vi "BSC simple.vi"() -> (0 "error out":errorcluster)   [LabVIEW 2016]
uses:
  C:/Users/Administrator/Downloads/LabVIEW/Kinesis/DLL Libraries/Thorlabs.MotionControl.Controls.dll
  DLL Libraries/Thorlabs.MotionControl.Controls.dll
  C:/Program Files (x86)/National Instruments/LabVIEW 2015/instr.lib/nLight Instruments/Motion Controller/Specific Models/Thorlabs Kinesis/Thorlabs.MotionControl.GenericMotorCLI.dll
  Program Files (x86)/National Instruments/LabVIEW 2015/instr.lib/nLight Instruments/Motion Controller/Specific Models/Thorlabs Kinesis/Thorlabs.MotionControl.GenericMotorCLI.dll
  C:/Program Files (x86)/National Instruments/LabVIEW 2015/instr.lib/nLight Instruments/Motion Controller/Specific Models/Thorlabs Kinesis/Thorlabs.MotionControl.Benchtop.StepperMotorCLI.dll
  Program Files (x86)/National Instruments/LabVIEW 2015/instr.lib/nLight Instruments/Motion Controller/Specific Models/Thorlabs Kinesis/Thorlabs.MotionControl.Benchtop.StepperMotorCLI.dll
panel:
  out "Position":dbl
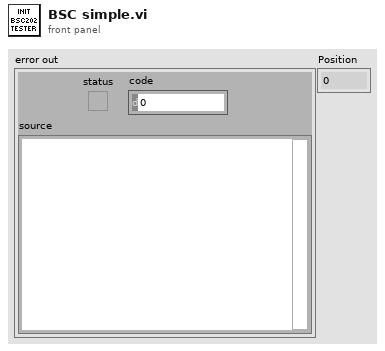
[diagram p1: front panel]
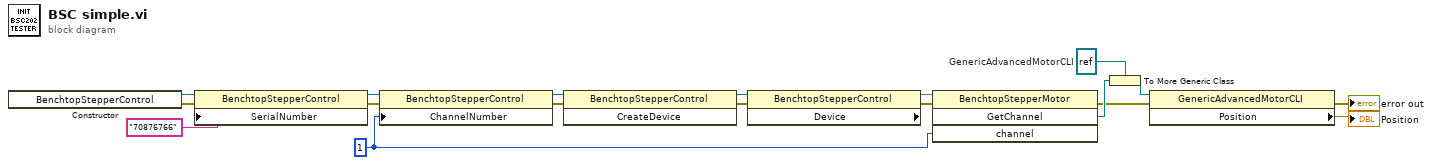
[diagram p0: block diagram]
diagram:
  w5 = i16 1 ("channel")
  w13 = refnum<k24> refnum  # GenericAdvancedMotorCLI
  n1 = constructor class="BenchtopStepperControl"() -> (reference out=w11:refnum<k24>, error out=w12:errorcluster)  [unwired: 3 in, 1 out]
  n2 = property class="BenchtopStepperControl"(reference=w11, error in=w12, "SerialNumber"="70876766") -> (reference out=w7:refnum<k24>, error out=w6:errorcluster)
  n3 = property class="BenchtopStepperControl"(reference=w7, error in=w6, "ChannelNumber"=w5) -> (reference out=w9:refnum<k24>, error out=w8:errorcluster)
  n4 = invoke class="BenchtopStepperControl" method="CreateDevice"(reference=w9, error in=w8) -> (reference out=w18:refnum<k24>, error out=w17:errorcluster)  [unwired: 1 in, 1 out]
  n5 = property class="BenchtopStepperControl"(reference=w18, error in=w17) -> (error out=w15:errorcluster, "Device"=w14)  [unwired: 1 out]
  n6 = invoke class="BenchtopStepperMotor" method="GetChannel"(reference=w14, error in=w15, "channel"=w5) -> (error out=w4:errorcluster, "GetChannel"=w10:refnum<k24>)  [unwired: 1 in, 2 out]
  n7 = To More Generic Class(target class=w13, reference=w10) -> (generic class reference=w3:refnum<k24>)
  n8 = property class="GenericAdvancedMotorCLI"(reference=w3, error in=w4) -> (error out=→"error out":errorcluster, "Position"=→"Position":dbl)  [unwired: 1 out]
